vi "Get Multiple.vi"(8 "error in (no error)":errorcluster, 10 "Names":string[](array[string]), 11 "Variables in":refnum<class "Variables.lvclass">) -> (0 "error out":errorcluster, 1 "Values":dbl[](array[numeric]), 2 "Not Found":bool, 3 "Variables out":refnum<class "Variables.lvclass">)   [LabVIEW 2020, in "VolatusSeq.lvlib" / "Variables.lvclass"]
uses:
  Variables.lvclass
  Variables.lvclass/Variables.ctl
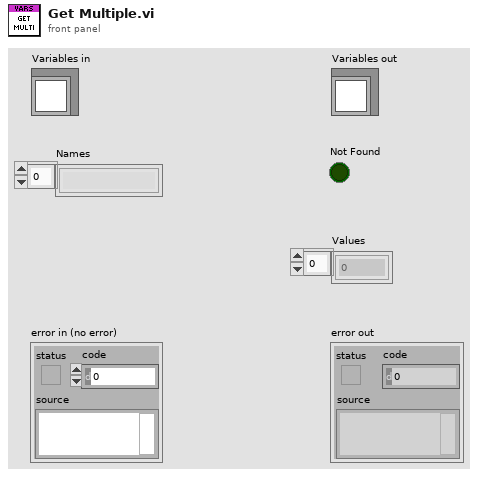
[diagram p1: front panel]
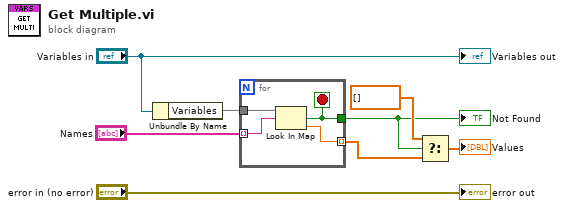
[diagram p0: block diagram]
diagram:
  n1 = Unbundle By Name("Variables in") -> ("Variables"=w6:map{string, dbl})
  n2 = for {
    tunnel: w6 -> [w12]
    tunnel: "Names" -> [w11] mode=indexing
    tunnel: [w10] -> w2
    tunnel: [w9] -> w4 mode=indexing
    stop <- w10 stop-if-true
    n3 = Look In Map(map=w12, key=w11) -> (key not found?=w10:bool, value=w9:dbl)  [unwired: 1 in]
  }
  "Not Found" <- w2
  n4 = Select(t=dbl[] [], s=w2, f=w4) -> (s? t:f=→"Values":dbl[])
  "error out" <- "error in (no error)"
  "Variables out" <- "Variables in"
